vi "Arm Globals.vi"() -> ()   [LabVIEW 2013]
uses:
  <vilib>/Analysis/Matrix/Datatypes/RealMatrix.ctl
  <vilib>/Analysis/Matrix/NI_Matrix.lvlib
panel:
  in  "Tab Control":enum32{"Main", "Right", "Left"}(tab)=enum."Right"
  in  "L:Pause":bool
  in  "L:End":bool
  out "L:Status":string="Home"
  in  "R:Pause":bool
  in  "R:End":bool
  out "R:Status":string="Safe"
  in  "Stop":bool
  in  "Configuration Path":path=path "C:/Program Files/Labview/user.lib/ROSforLV_0.1/Devices/Baxter/Cartesian/Object Locations.ini"
  in  "R:Units":string="mm"
  in  "R:Speed":dbl=25.0 format="%.1f"
  in  "R:Jt Limits":dbl[][](array[numeric])=[[51.0, -141.0], [60.0, -123.0], [173.5, -173.5], [150.0, -3.0], [175.25, -175.25], [120.0, -90.0], [175.25, -175.25]] format="%.2f"
  in  "R: Left of Post":dbl[](array[numeric])=[1.0, -80.0, 0.0, 120.0, 0.0, 50.0, 0.0] format="%.3f"
  in  "R: Right of Post":dbl[](array[numeric])=[-1.0, -80.0, 0.0, 120.0, 0.0, 50.0, 0.0] format="%.3f"
  in  "R:Command":cluster{"Label":string, "Angles":dbl[]}={"Label"="Safe", "Angles"=[-40.0, -65.0, 0.0, 90.0, 0.0, 65.0, 0.0]} {"Angles" format="%.3f"}
  in  "R:tTg":T1=[[-1.0, 0.0, 0.0, 0.0], [0.0, 1.0, 0.0, 0.0], [0.0, 0.0, -1.0, 99.0], [0.0, 0.0, 0.0, 1.0]] caption="Tool plate to gripper point"
  in  "R:tTc":T1=[[-1.0, 0.0, 0.0, 40.0], [0.0, 1.0, 0.0, 12.0], [0.0, 0.0, -1.0, 0.0], [0.0, 0.0, 0.0, 1.0]] caption="Tool plate to Camera"
  in  "L:Jt Limits":dbl[][](array[numeric])=[[141.0, -51.0], [60.0, -123.0], [173.5, -173.5], [150.0, -3.0], [175.25, -175.25], [120.0, -90.0], [175.25, -175.25]] format="%.2f"
  in  "L: Left of Post":dbl[](array[numeric])=[0.0, -80.0, 0.0, 150.0, 0.0, 20.0, 0.0] format="%.3f"
  in  "L: Right of Post":dbl[](array[numeric])=[-25.0, -80.0, 0.0, 150.0, 0.0, 20.0, 0.0] format="%.3f"
  in  "L:Command":cluster{"Label":string, "Angles":dbl[]}={"Label"="", "Angles"=[0.0, -80.0, 0.0, 150.0, 0.0, 20.0, 0.0]} {"Angles" format="%.3f"}
  in  "L:tTg":T1=[[-1.0, 0.0, 0.0, 0.0], [0.0, 1.0, 0.0, 0.0], [0.0, 0.0, -1.0, 99.0], [0.0, 0.0, 0.0, 1.0]] caption="Tool plate to gripper point"
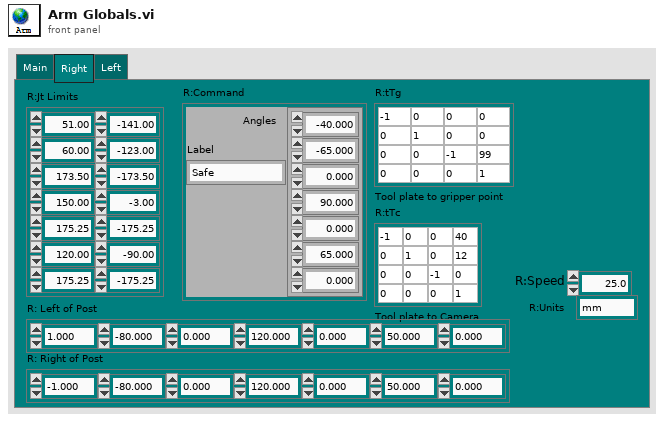
[diagram p1: front panel]
types:
  T1 = typedef "NI_Matrix.lvlib/RealMatrix.ctl" = dbl[][]
diagram:
